vi "motor_example_noarduino.vi"() -> ()   [LabVIEW 2014]
uses:
  statecontrol.ctl
panel:
  out "Tab Control":enum32{" On", "Off", "CoolDown"}(tab)
  in  "On":bool
  in  "Off":bool
  out "Cooldown":bool
  out "millisecond timer value 4":u32
  out "Cooldown Time Left 2":u32
  in  "set superlight on timer [ms]":u32
  out "superlight status":bool
  out "millisecond timer value 2":u32
  in  "stop":bool
  out "Cooldown Time Left":u32 format="%<%M:%S>t"
  out "cooldown status":bool
  in  "set cooldown timer [ms]":u32
  in  "index pulse":bool
  out "state":T1
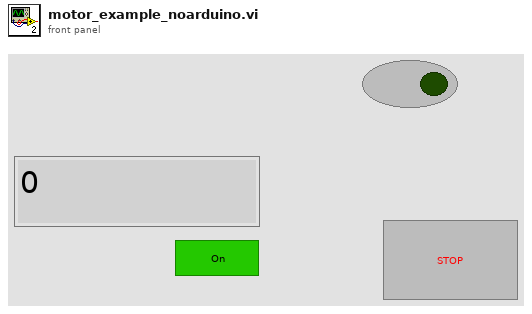
[diagram p1: front panel]
types:
  T1 = typedef "statecontrol.ctl" = enum16{"init", "waiting for trigger", "superlight on", "cooldown", "shutdown"}
  T2 = enum8{"Enabled", "Disabled", "Disabled and Grayed Out"}
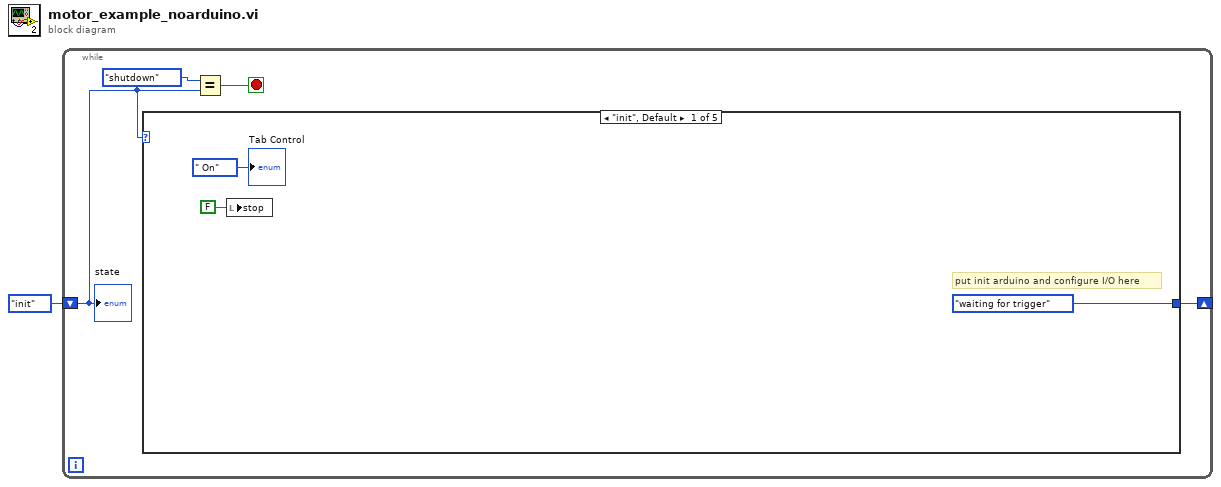
[diagram p0: block diagram]
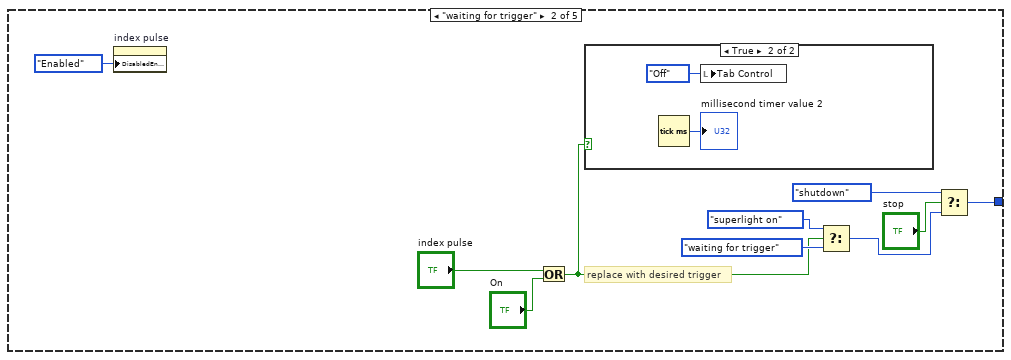
[diagram p2: hidden frame]
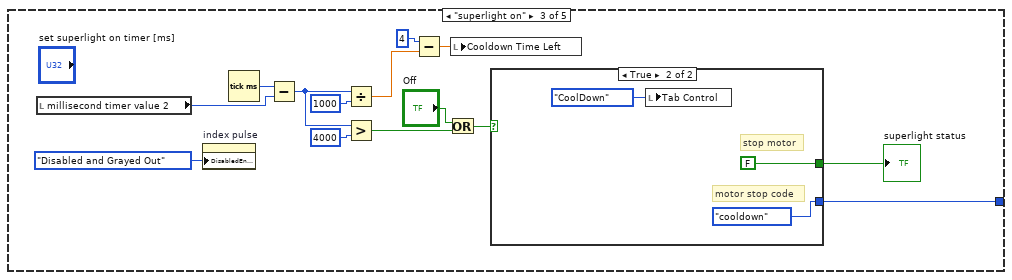
[diagram p4: hidden frame]
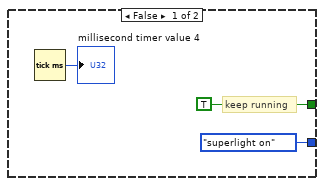
[diagram p5: hidden frame]
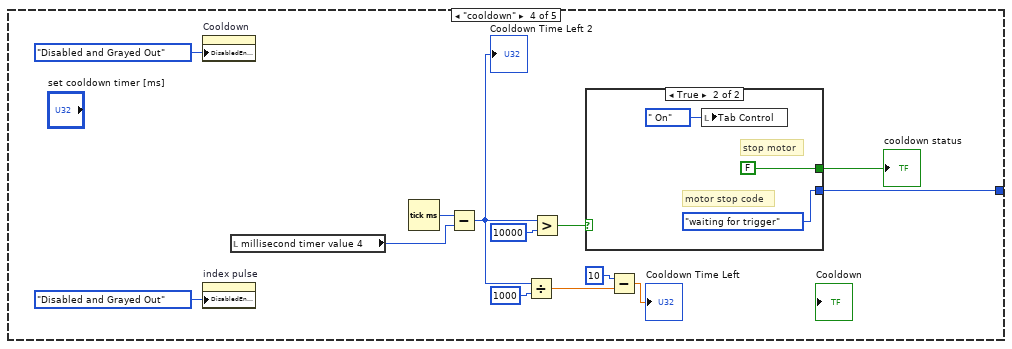
[diagram p6: hidden frame]
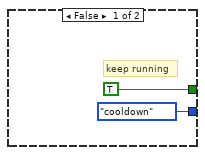
[diagram p7: hidden frame]
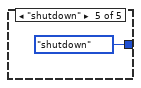
[diagram p8: hidden frame]
diagram:
  n1 = while {
    shift-right: [w2] -> _
    shift-left: statecontrol."init" ("state") -> [w3]
    stop <- w4 stop-if-true
    n2 = case shown="\"init\", Default" w3 {
      tunnel: [statecontrol."waiting for trigger" ("state") w13 w31 w49 statecontrol."shutdown" ("state")] -> w2
      frame "init", Default {
        # "put init arduino and configure I/O here"
        n3 = local write "stop"(FALSE ("stop")) -> ()
        "Tab Control" <- enum32{" On", "Off", "CoolDown"}." On" ("Tab Control")
      }
      frame "waiting for trigger" {
        # "replace with desired trigger"
        n4 = property on="index pulse" class="Bool"("DisabledEnum"=T2."Enabled" ("Disabled")) -> ()  [unwired: 2 in, 2 out]
        n5 = Or(x="index pulse", y="On") -> (x .or. y?=w9:bool)
        n6 = case shown="True" w9 {
          frame False {
          }
          frame True {
            n7 = Tick Count (ms)() -> (millisecond timer value=→"millisecond timer value 2":u32)
            n8 = local write "Tab Control"(enum32{" On", "Off", "CoolDown"}."Off" ("Tab Control")) -> ()
          }
        }
        n9 = Select(t=statecontrol."superlight on" ("state"), s=w9, f=statecontrol."waiting for trigger" ("state")) -> (s? t:f=w14:T1)
        n10 = Select(t=statecontrol."shutdown" ("state"), s="stop", f=w14) -> (s? t:f=w13:T1)
      }
      frame "superlight on" {
        n11 = local read "millisecond timer value 2"() -> (w34:u32)
        n12 = property on="index pulse" class="Bool"("DisabledEnum"=T2."Disabled and Grayed Out" ("Disabled")) -> ()  [unwired: 2 in, 2 out]
        n13 = Tick Count (ms)() -> (millisecond timer value=w33:u32)
        n14 = Subtract(x=w33, y=w34) -> (x-y=w29:u32)
        n15 = Divide(x=w29, y=u32 1000) -> (x/y=w27:dbl)
        n16 = Greater?(x=w29, y=u32 4000) -> (0:w23:bool)
        n17 = Subtract(x=u32 4, y=w27) -> (x-y=w21:dbl)
        n18 = Or(x="Off", y=w23) -> (x .or. y?=w22:bool)
        n19 = local write "Cooldown Time Left"(w21) -> ()
        n20 = case shown="True" w22 {
          tunnel: [TRUE FALSE] -> w32
          tunnel: [statecontrol."superlight on" ("state") statecontrol."cooldown" ("state")] -> w31
          frame False {
            # "keep running"
            n21 = Tick Count (ms)() -> (millisecond timer value=→"millisecond timer value 4":u32)
          }
          frame True {
            # "motor stop code"
            # "stop motor"
            n22 = local write "Tab Control"(enum32{" On", "Off", "CoolDown"}."CoolDown" ("Tab Control")) -> ()
          }
        }
        "superlight status" <- w32
      }
      frame "cooldown" {
        n23 = property on="Cooldown" class="Bool"("DisabledEnum"=T2."Disabled and Grayed Out" ("Disabled")) -> ()  [unwired: 2 in, 2 out]
        n24 = property on="index pulse" class="Bool"("DisabledEnum"=T2."Disabled and Grayed Out" ("Disabled")) -> ()  [unwired: 2 in, 2 out]
        n25 = local read "millisecond timer value 4"() -> (w53:u32)
        n26 = Tick Count (ms)() -> (millisecond timer value=w52:u32)
        n27 = Subtract(x=w52, y=w53) -> (x-y=w45:u32)
        "Cooldown Time Left 2" <- w45
        n28 = Divide(x=w45, y=u32 1000) -> (x/y=w46:dbl)
        n29 = Greater?(x=w45, y=u32 10000) -> (0:w51:bool)
        n30 = case shown="True" w51 {
          tunnel: [TRUE FALSE] -> w50
          tunnel: [statecontrol."cooldown" ("state") statecontrol."waiting for trigger" ("state")] -> w49
          frame False {
            # "keep running"
          }
          frame True {
            # "motor stop code"
            # "stop motor"
            n31 = local write "Tab Control"(enum32{" On", "Off", "CoolDown"}." On" ("Tab Control")) -> ()
          }
        }
        "cooldown status" <- w50
        n32 = Subtract(x=u32 10, y=w46) -> (x-y=→"Cooldown Time Left":dbl)
      }
      frame "shutdown" {
      }
    }
    n33 = Equal?(x=statecontrol."shutdown" ("state"), y=w3) -> (x = y?=w4:bool)
    "state" <- w3
  }
